vi "NF WF1973_74 SEQ Stor.vi"(5 "Name(USERNAME)":string="USERNAME", 7 "File No.(1)":i32=1 min=1 max=10 step=1, 8 "error in (no error)":errorcluster caption="Error IN", 11 "VISAsession":refnum<visa-resource-name>) -> (0 "error out":errorcluster caption="Error OUT", 3 "CopyVISAsession":refnum<visa-resource-name>)   [LabVIEW 2010]
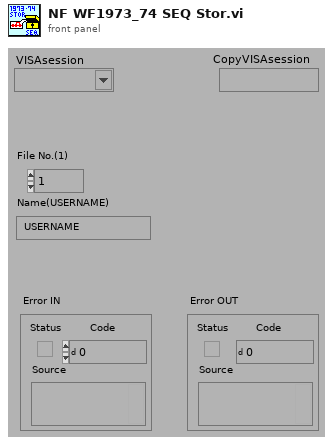
[diagram p1: front panel]
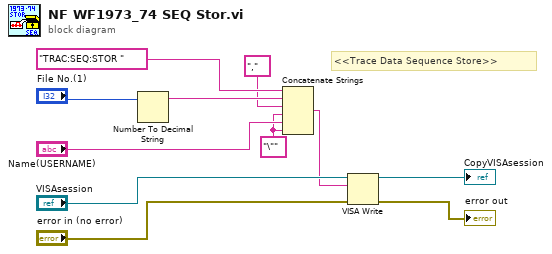
[diagram p0: block diagram]
diagram:
  w1 = "\""
  # "<<Trace Data Sequence Store>>"
  n1 = Number To Decimal String(number="File No.(1)") -> (decimal integer string=w5:string)  [unwired: 1 in]
  n2 = Concatenate Strings("TRAC:SEQ:STOR ", w5, ",", w1, "Name(USERNAME)", w1) -> (w4:string)
  n3 = VISA Write(VISA resource name="VISAsession", write buffer=w4, error in (no error)="error in (no error)") -> (VISA resource name out=→"CopyVISAsession":refnum<visa-resource-name>, error out=→"error out":errorcluster)  [unwired: 1 out]
